vi "Action executor.vi"(7 "Action":T1, 11 "error in (no error)":errorcluster) -> (6 "Stop Motor":bool, 8 "P 3.Stop Motor Voltage":dbl, 15 "error out":errorcluster)   [LabVIEW 2011]
uses:
  Action List.ctl
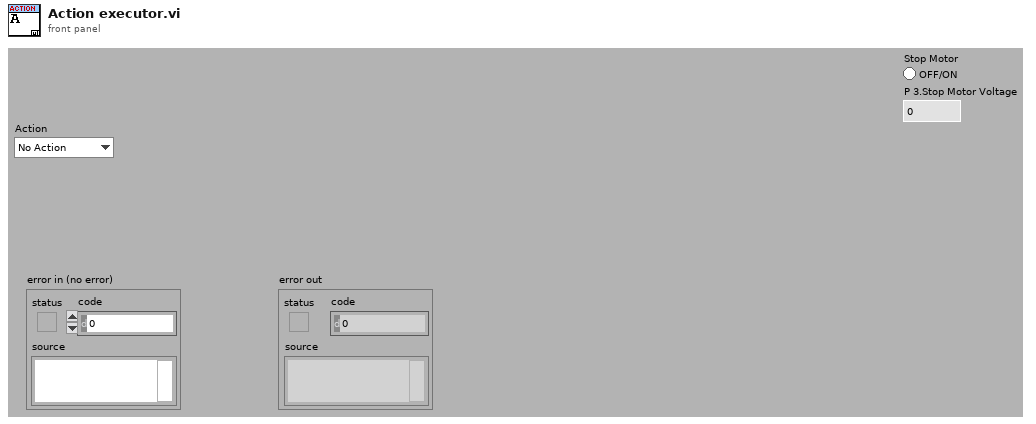
[diagram p1: front panel]
types:
  T1 = typedef "Action List.ctl" = enum16{"No Action", "Stop Motor", "Turn Off HV"}
  T2 = typedef "Options  All pages and custom.ctl" = cluster{"P 1 (App)":T3, "P 2":T4, "P 3":T5, "P 4":T8, "P 5":T13, "P 6 (Err)":T14, "P 7 (Expert)":T15, "P 8 (Depth)":T17, "C 1":T18, "C 2":T19}
  T3 = typedef "Options Page 1 (App).ctl" = cluster{"Result files":path, "PCP Interface":string, "Tractor/Stroker Interface":string, "Tractor Interface":string, "Modem Status Interface":string, "Audible Alarm":bool, "Force alarm on Technical":bool, "Force alarm on HH":bool, "Force alarm on LL":bool, "Force alarm on H":bool, "Force alarm on L":bool}
  T4 = typedef "Options Page 2.ctl" = cluster{"Solenoid & Relay latching time":u16, "Tractor relay 1":dbl, "Tractor relay 2":dbl, "Tractor Solenoid limit":dbl}
  T5 = typedef "Options Page 3.ctl" = cluster{"Min resistance":dbl, "Max resistance":dbl, "Head voltage range":T6, "Max voltage jump":dbl, "Maximum resistance change":dbl, "Start Telemetry Voltage":dbl, "Start Telemetry Timeout":dbl, "Start Motor Voltage":dbl, "Stop Motor Voltage":dbl, "Pass Mode Warning Voltage":dbl, "Relay Switch Voltage":dbl, "Relay Status Loss Voltage":dbl, "Samples to average":i32, "PSU type DO NOT USE":T7, "Magna OVP":dbl, "Magna Current Limit":dbl}
  T6 = typedef "PCP type List.ctl" = enum16{"0 - 350V", "0 - 450V", "0 - 600V"}
  T7 = typedef "PSU Type.ctl" = enum16{"Unipower", "Magna 8.3A", "Magna 12A", "None"}
  T8 = typedef "Options Page 4.ctl" = cluster{"Solenoid & Relay latching time":u16, "Stroker relay 1":dbl, "Stroker Relay 2":dbl, "Stroker Solenoid limit":dbl, "Force det.":T9, "Stroke force lim.":dbl, "Anchor Enabled Pressure":dbl, "Tacometer puls":dbl, "Default anchor behavior":T10, "Default stroker behavior":T11, "Default stroker force limit (tonne)":dbl, "Slips Size":T12}
  T9 = typedef "Stroke force selector.ctl" = enum16{"Stroke in = node 1", "Strok out = node 1"}
  T10 = typedef "Default anchor behavior.ctl" = enum16{"Do nothing", "Set Anchor", "Release Anchor"}
  T11 = typedef "Default stroker behavior.ctl" = enum16{"Do nothing", "Stop", "Go Out", "Go In"}
  T12 = typedef "Slips Type Radio.ctl" = enum32{"No Selection", "338 MRS", "3,9 MRS"}
  T13 = typedef "Options Page 5.ctl" = cluster{"Solenoid & Relay latching time":u16, "Driller relay 1":dbl, "Driller Relay 2":dbl, "Driller  Solenoid limit":dbl}
  T14 = typedef "Options Page 6 (Err).ctl" = cluster{"Error and event files":path}
  T15 = typedef "Options Page 7 (Expert).ctl" = cluster{"Show Debug":bool, "Log debug messages":bool, "Additional debug messages":bool, "Start Beagle with Simulator data":bool, "Workshop mode":bool, "Modem baud":u16, "enumCANCOM":bool, "Modem sim":T16, "Telemetry Timeout Disable":i32, "Buffer size":i32, "Upd regular data":bool, "Cable comp":cluster{"VMOD1 Voltage(V)":dbl, "VMOD2 Voltage(V)":dbl}}
  T16 = typedef "Modem simulation setup.ctl" = cluster{"Modem dealay sim":bool, "Sim baud Tx":u16, "Bit Error fraction Tx":dbl, "Sim baud Rx":u16, "Bit Error fraction Rx":dbl}
  T17 = typedef "Options Page 8 (Depth).ctl" = cluster{"Winch Spool Circumference":dbl, "Winch Pulses per Revolution":dbl, "Current Depth":dbl}
  T18 = typedef "Options Custom 1.ctl" = cluster{"Depth Updated":bool, "Depth Offset":dbl}
  T19 = typedef "Options Custom 2.ctl" = cluster{"Placeholder":bool}
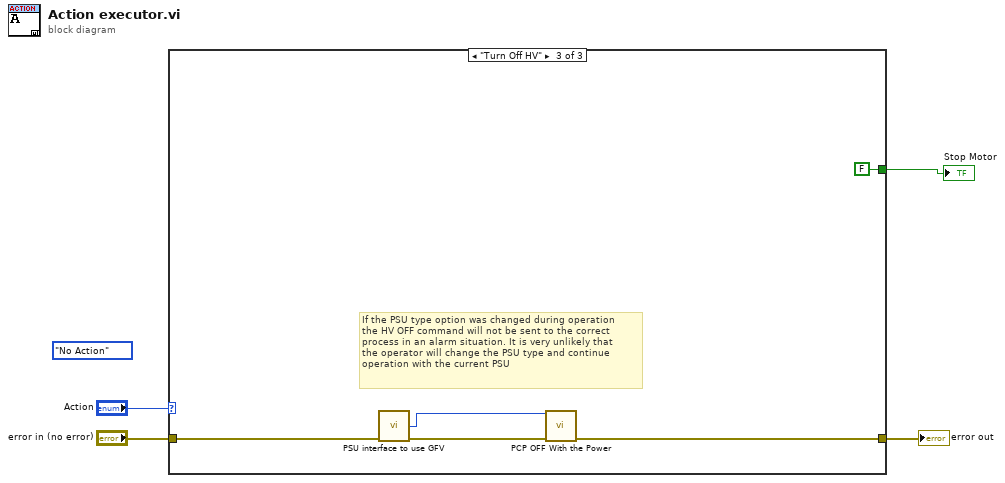
[diagram p0: block diagram]
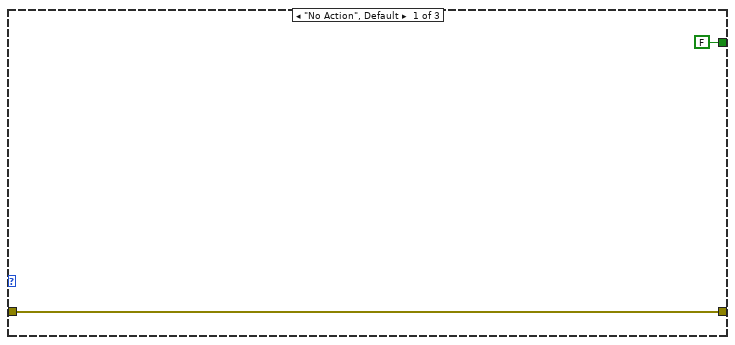
[diagram p2: hidden frame]
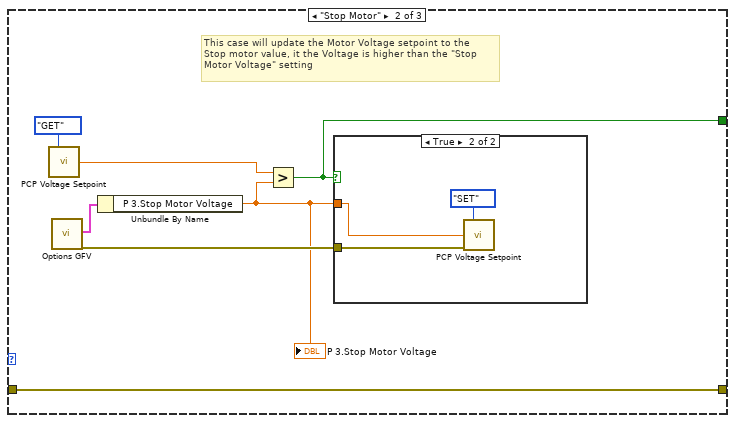
[diagram p3: hidden frame]
diagram:
  (unwired) Action_List."No Action" ("Action 2")
  n1 = case shown="\"Turn Off HV\"" "Action" {
    tunnel: "error in (no error)" -> [w6 w13 w19]
    tunnel: [w6 w13 w21] -> w2
    tunnel: [FALSE w9 FALSE] -> w1
    frame "No Action", Default {
    }
    frame "Stop Motor" {
      # "This case will update the Motor Voltage setpoint to the \nStop motor value, it the Voltage is higher than the \"Stop\nMotor Voltage\" setting"
      n2 = call "PCP Voltage Setpoint.vi"("Action(GET)"=enum16{"GET", "SET"}."GET") -> ("PCP setpoint"=w8:dbl)  [unwired: 13 in, 1 out]
      n3 = call "Options GFV.vi"() -> ("Options"=w11:T2, "error out"=w12:errorcluster)  [unwired: 17 in, 1 out]
      n4 = Unbundle By Name(w11) -> ("P 3.Stop Motor Voltage"=w7:dbl)
      "P 3.Stop Motor Voltage" <- w7
      n5 = Greater?(x=w8, y=w7) -> (0:w9:bool)
      n6 = case shown="True" w9 {
        tunnel: w12 -> [_ w16]
        tunnel: w7 -> [_ w14]
        frame False {
        }
        frame True {
          n7 = call "PCP Voltage Setpoint.vi"("Action(GET)"=enum16{"GET", "SET"}."SET", "PCP HV setpoint"=w14, "error in (no error)"=w16) -> ()  [unwired: 11 in, 2 out]
        }
      }
    }
    frame "Turn Off HV" {
      # "If the PSU type option was changed during operation\nthe HV OFF command will not be sent to the correct\nprocess in an alarm situation. It is very unlikely that\nthe operator will change the PSU type and continue \noperation with the current PSU"
      n8 = call "PSU interface to use GFV.vi"("error in (no error)"=w19) -> ("PSU type  out"=w17:T7, "error out"=w18:errorcluster)  [unwired: 13 in]
      n9 = call "PCP OFF With the Power.vi"("PSU type"=w17, "error In"=w18) -> ("error out"=w21:errorcluster)  [unwired: 13 in]
    }
  }
  "error out" <- w2
  "Stop Motor" <- w1
